vi "server.vi"() -> ()   [LabVIEW 2021]
panel:
  in  "Indirizzo IP":string
  out "Frequenza non trovata":bool
  out "Costante step variabile":dbl
  out "Freq -3dB":dbl
  out "Vpp=Vout":dbl
  out "Vrms=Vin":dbl
  out "V zero-picco":dbl
  out "Frequenza corrente":dbl
  out "Indice misurazione corrente":i32
  out "Comando ampiezza":string
  out "Vpp":string
  in  "Indirizzo Multimetro":string
  out "Comando frequenza":string
  out "f_stop":string
  out "Ampiezza":string
  out "Step di frequenza":string
  out "f_start":string
  out "Password":string
  out "Array":string[](array[string])
  in  "Porta":u16
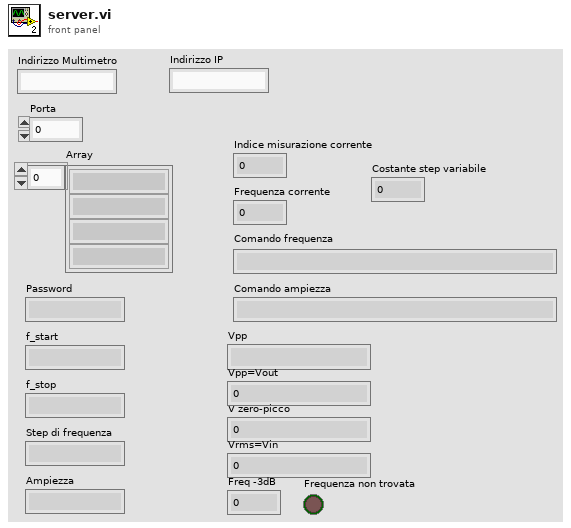
[diagram p1: front panel]
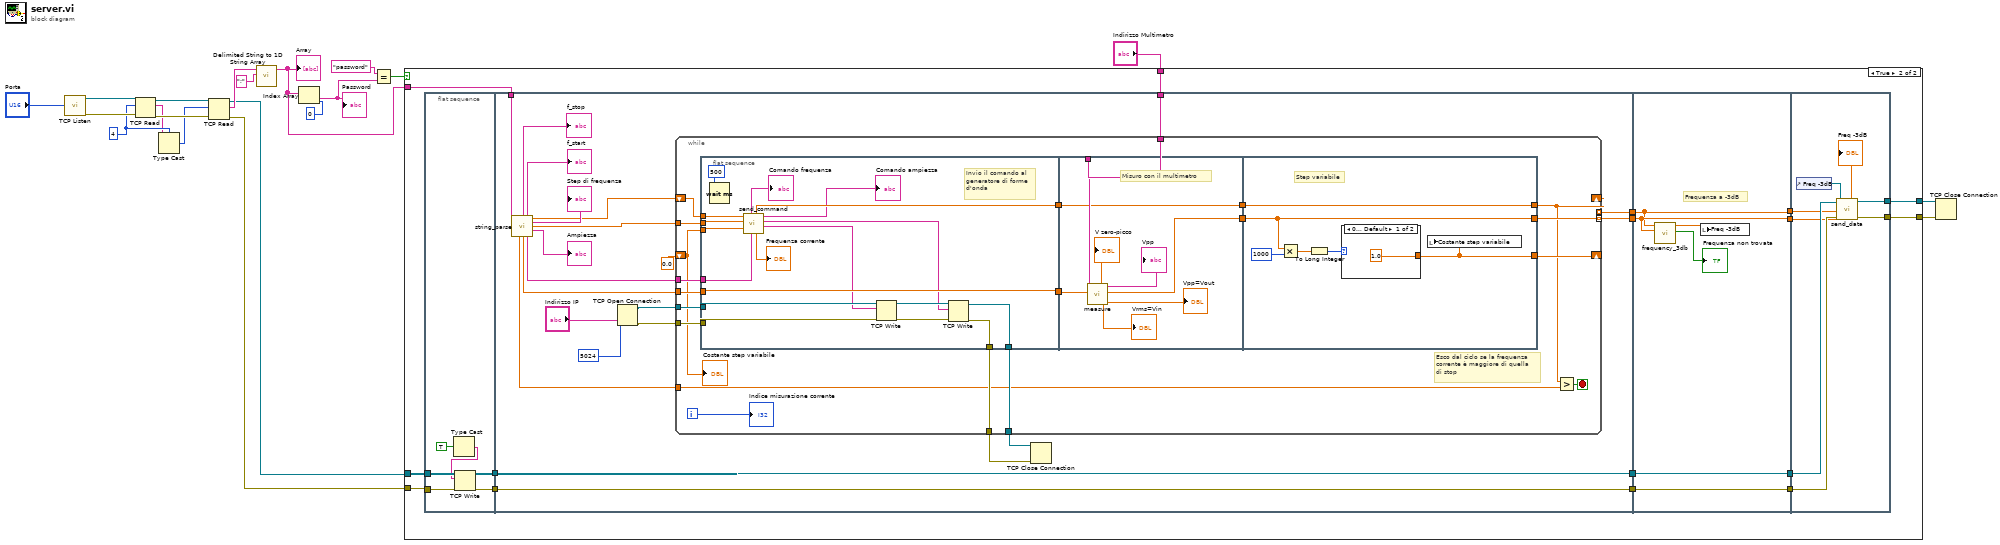
[diagram p0: block diagram]
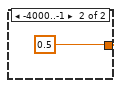
[diagram p3: hidden frame]
diagram:
  w15 = 4 ("bytes to read")
  n1 = call <vilib>:"TCP Listen.vi"("port"="Porta") -> ("error out"=w17:errorcluster, "connection ID"=w19:refnum<k5>)  [unwired: 6 in, 3 out]
  n2 = TCP Read(connection ID=w19, bytes to read=w15, error in (no error)=w17) -> (connection ID out=w18:refnum<k5>, data out=w14:string, error out=w16:errorcluster)  [unwired: 2 in]
  n3 = Type Cast(type=w15, x=w14) -> (*(type *) &x=w13:i32)
  n4 = TCP Read(connection ID=w18, bytes to read=w13, error in (no error)=w16) -> (connection ID out=w7:refnum<k5>, data out=w11:string, error out=w6:errorcluster)  [unwired: 2 in]
  n5 = call <vilib>:"Delimited String to 1D String Array.vi"("delimiter"=";" ("delimiter (Tab)"), "delimited string"=w11) -> ("string array"=w1:string[])  [unwired: 9 in]
  "Array" <- w1
  n6 = Index Array(array=w1, index=0) -> (element=w4:string)
  "Password" <- w4
  n7 = Equal?(x="password", y=w4) -> (x = y?=w8:bool)
  n8 = case shown="True" w8 {
    tunnel: w1 -> [_ w35]
    tunnel: w7 -> [w22 w37]
    tunnel: w6 -> [w21 w38]
    tunnel: "Indirizzo Multimetro" -> [_ w36]
    tunnel: [w22 w32] -> w2
    tunnel: [w21 w31] -> w3
    frame False {
    }
    frame True {
      n9 = flat-sequence {
        tunnel: w38 -> [w42]
        tunnel: w37 -> [w41]
        tunnel: [w40] -> w34
        tunnel: [w39] -> w33
        tunnel: w36 -> [w66]
        tunnel: w35 -> [w65]
        tunnel: w34 -> [w63]
        tunnel: w33 -> [w64]
        tunnel: [w64] -> w30
        tunnel: [w63] -> w28
        tunnel: [w62] -> w26
        tunnel: [w61] -> w24
        tunnel: w30 -> [w126]
        tunnel: [w126] -> w29
        tunnel: w28 -> [w125]
        tunnel: [w125] -> w27
        tunnel: w26 -> [w124]
        tunnel: [w124] -> w25
        tunnel: w24 -> [w123]
        tunnel: [w123] -> w23
        tunnel: w29 -> [w134]
        tunnel: w27 -> [w133]
        tunnel: w25 -> [w132]
        tunnel: w23 -> [w131]
        tunnel: [w130] -> w32
        tunnel: [w129] -> w31
        frame #0 {
          n10 = Type Cast(x=TRUE) -> (*(type *) &x=w44:string)  [unwired: 1 in]
          n11 = TCP Write(connection ID=w41, data in=w44, error in (no error)=w42) -> (connection ID out=w40:refnum<k5>, error out=w39:errorcluster)  [unwired: 1 in, 1 out]
        }
        frame #1 {
          n12 = call "string_parse.vi"("string array"=w65) -> ("f_stop"=→"f_stop":string, "f_start"=→"f_start":string, "f_start double"=w50:dbl, "Step di frequenza"=→"Step di frequenza":string, "Step di frequenza double"=w46:dbl, "Ampiezza"=→"Ampiezza":string, "f_stop double"=w47:dbl, "Ampiezza double"=w48:dbl, "Ampiezza string"=w49:string)  [unwired: 6 in]
          n13 = TCP Open Connection(address="Indirizzo IP", remote port or service name=u16 5024) -> (connection ID=w60:refnum<k5>, error out=w59:errorcluster)  [unwired: 3 in]
          n14 = while {
            tunnel: w49 -> [w86]
            tunnel: w46 -> [w85]
            tunnel: w66 -> [w84]
            tunnel: w60 -> [w83]
            tunnel: w59 -> [w82]
            tunnel: [w81] -> w57
            tunnel: [w80] -> w56
            tunnel: w48 -> [w78]
            tunnel: [w68] -> w61 mode=indexing
            tunnel: [w76] -> w62 mode=indexing
            tunnel: w47 -> [w75]
            shift-right: [w72] -> _
            shift-left: 0.0 -> [w71]
            shift-right: [w68] -> _
            shift-left: w50 -> [w67]
            i -> [w70]
            stop <- w69 stop-if-true
            # "Esco dal ciclo se la frequenza\ncorrente è maggiore di quella\ndi stop"
            n15 = flat-sequence {
              tunnel: w86 -> [w103]
              tunnel: w85 -> [w95]
              tunnel: w83 -> [w101]
              tunnel: w82 -> [w100]
              tunnel: [w97] -> w81
              tunnel: [w96] -> w80
              tunnel: [w91] -> w79
              tunnel: w78 -> [w102]
              tunnel: [w102] -> w77
              tunnel: w71 -> [w94]
              tunnel: w67 -> [w93]
              tunnel: w84 -> [w112]
              tunnel: w79 -> [w110]
              tunnel: w77 -> [w111]
              tunnel: [w110] -> w74
              tunnel: [w109] -> w73
              tunnel: [w113] -> w76
              tunnel: [w118] -> w68
              tunnel: w74 -> [w118]
              tunnel: w73 -> [w113]
              tunnel: [w114] -> w72
              frame #0 {
                # "Invio il comando al generatore di forme d'onda"
                n16 = Wait (ms)(milliseconds to wait=u32 500) -> ()  [unwired: 1 out]
                n17 = call "send_command.vi"("Ampiezza"=w103, "Step in frequenza"=w94, "Costante"=w95, "f_start"=w93) -> ("out Comando frequenza"=w88:string, "out Comando ampiezza"=w87:string, "Comando ampiezza"=→"Comando ampiezza":string, "Frequenza corrente"=→"Frequenza corrente":dbl, "out Frequenza corrente"=w91:dbl, "Comando frequenza"=→"Comando frequenza":string)  [unwired: 2 in]
                n18 = TCP Write(connection ID=w101, data in=w88, error in (no error)=w100) -> (connection ID out=w99:refnum<k5>, error out=w98:errorcluster)  [unwired: 1 in, 1 out]
                n19 = TCP Write(connection ID=w99, data in=w87, error in (no error)=w98) -> (connection ID out=w97:refnum<k5>, error out=w96:errorcluster)  [unwired: 1 in, 1 out]
              }
              frame #1 {
                # "Misuro con il multimetro"
                n20 = call "measure.vi"("Ampiezza"=w111, "Indirizzo Multimetro"=w112) -> ("Vpp=Vout"=→"Vpp=Vout":dbl, "(Vout/Vin)dB"=w109:dbl, "Vpp"=→"Vpp":string, "Vrms=Vin"=→"Vrms=Vin":dbl, "V zero-picco"=→"V zero-picco":dbl)  [unwired: 5 in]
              }
              frame #2 {
                # "Step variabile"
                n21 = Multiply(x=w113, y=1000) -> (x*y=w116:dbl)
                n22 = To Long Integer(number=w116) -> (32bit integer=w117:i32)
                n23 = case shown="0.., Default" w117 {
                  tunnel: [1.0 0.5] -> w114
                  frame 0.., Default {
                  }
                  frame -4000..-1 {
                  }
                }
                n24 = local write "Costante step variabile"(w114) -> ()
              }
            }
            n25 = Greater?(x=w68, y=w75) -> (0:w69:bool)
            "Indice misurazione corrente" <- w70
            "Costante step variabile" <- w71
          }
          n26 = TCP Close Connection(connection ID=w57, error in (no error)=w56) -> ()  [unwired: 1 in, 2 out]
        }
        frame #2 {
          # "Frequenza a -3dB"
          n27 = call "frequency_3db.vi"("Misure"=w124, "Frequenze"=w123) -> ("Frequenza non trovata"=→"Frequenza non trovata":bool, "Frequenza -3dB"=w122:dbl)  [unwired: 8 in]
          n28 = local write "Freq -3dB"(w122) -> ()
        }
        frame #3 {
          n29 = control-ref of="Freq -3dB"() -> (w128:refnum<vi>)
          n30 = call "send_data.vi"("Misure"=w132, "error in (no error)"=w134, "Frequenze"=w131, "connection ID in"=w133, "Digital in"=w128) -> ("error out"=w129:errorcluster, "Freq -3dB"=→"Freq -3dB":dbl, "TCP Network Connection out"=w130:refnum<k5>)  [unwired: 4 in]
        }
      }
    }
  }
  n31 = TCP Close Connection(connection ID=w2, error in (no error)=w3) -> ()  [unwired: 1 in, 2 out]
